vi "Custom Drive.vi"(8 "error in (no error)":errorcluster, 9 "RightSpeed":dbl, 10 "LeftSpeed":dbl, 11 "RobotDriveDevRef":T1={"DevStatus"={"status"=FALSE, "code"=0, "source"=""}, "Motors[]"=[], "Square Inputs"=FALSE, "Max Output"=1.0}) -> (0 "error out":errorcluster, 2 "Motor Values":dbl[](array[numeric]), 3 "RobotDriveDevRef":T1={"DevStatus"={"status"=FALSE, "code"=0, "source"=""}, "Motors[]"=[], "Square Inputs"=FALSE, "Max Output"=1.0})   [LabVIEW 2015]
doc: "Determines the motor configuration and sends the speed values to the appropriate motors.\n\nThis software is licensed. Open the labview\\readme\\WPI Robotics Library Open Source License.txt file for more information."
uses:
  <vilib>/Rock Robotics/WPI/RobotDrive/WPI_RobotDriveDevRef.ctl
  <vilib>/Rock Robotics/WPI/MotorControl/WPI_MotorControlDeviceRef.ctl
  <vilib>/Rock Robotics/WPI/MotorControl/WPI_MotorControlType.ctl
  <vilib>/Rock Robotics/SystemInterfaces/DIO/FPGA_DIOPWMChannel.ctl
  <vilib>/Rock Robotics/WPI/PWM/WPI_PWMDeadband.ctl
  <vilib>/Rock Robotics/WPI/CAN/Jaguar/SubVIs/WPI_CANJaguar_ControlMode.ctl
  <vilib>/Rock Robotics/WPI/CAN/TalonSRX/WPI_CANTalonSRX_APIControlMode.ctl
  <vilib>/Rock Robotics/WPI/RobotDrive/WPI_RobotDriveSafetyCheck.vi
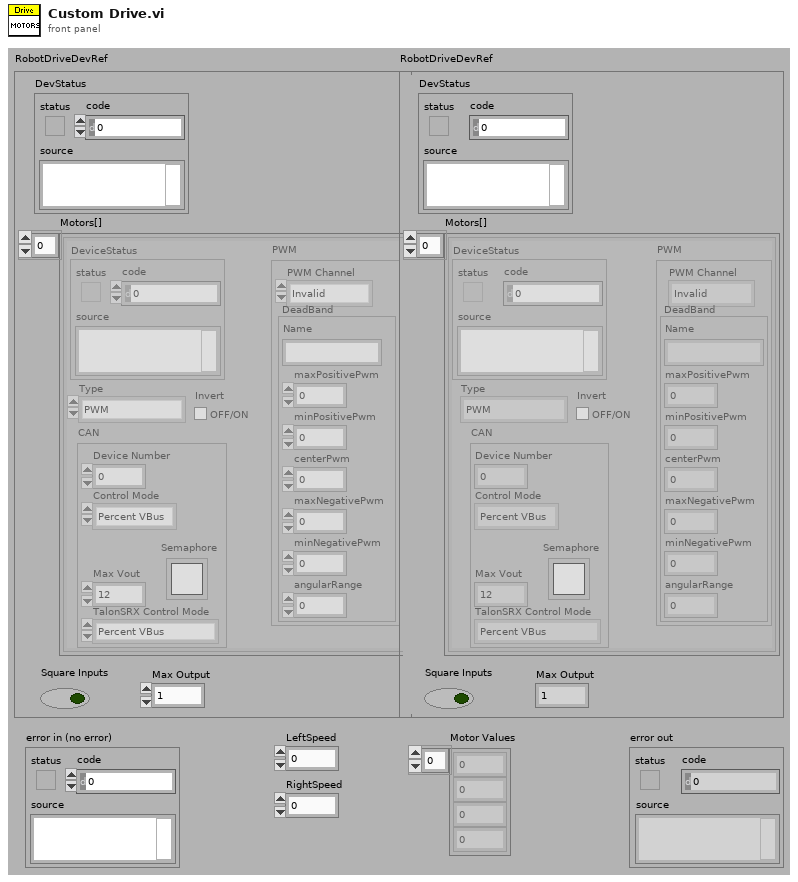
[diagram p1: front panel]
types:
  T1 = typedef "WPI_RobotDriveDevRef.ctl" = cluster{"DevStatus":errorcluster, "Motors[]":T2[], "Square Inputs":bool, "Max Output":dbl}
  T2 = typedef "WPI_MotorControlDeviceRef.ctl" = cluster{"DeviceStatus":errorcluster, "Type":T3, "PWM":cluster{"PWM Channel":T4, "DeadBand":T5}, "CAN":cluster{"Device Number":u8, "Control Mode":T6, "Semaphore":T7, "Max Vout":dbl, "TalonSRX Control Mode":T8}, "Invert":bool}
  T3 = typedef "WPI_MotorControlType.ctl" = enum16{"PWM", "CAN", "CANTalonSRX"}
  T4 = typedef "FPGA_DIOPWMChannel.ctl" = enum8{"PWM 0", "PWM 1", "PWM 2", "PWM 3", "PWM 4", "PWM 5", "PWM 6", "PWM 7", "PWM 8", "PWM 9", "PWM MXP 0", "PWM MXP 1", "PWM MXP 2", "PWM MXP 3", "PWM MXP 4", "PWM MXP 5", "PWM MXP 6", "PWM MXP 7", "PWM MXP 8", "PWM MXP 9", "Invalid"}
  T5 = typedef "WPI_PWMDeadband.ctl" = cluster{"Name":string, "maxPositivePwm":i32, "minPositivePwm":i32, "centerPwm":i32, "maxNegativePwm":i32, "minNegativePwm":i32, "angularRange":u16}
  T6 = typedef "WPI_CANJaguar_ControlMode.ctl" = enum8{"Percent VBus", "Current", "Speed", "Position", "Voltage"}
  T7 = typedef "Semaphore RefNum" = refnum<k1>
  T8 = typedef "WPI_CANTalonSRX_APIControlMode.ctl" = enum8{"Percent VBus", "Speed", "Position", "Slave", "Unchanged / Invalid", "Voltage Compensation", "Current", "Motion Profile"}
  T9 = enum16{"Rear Left Motor", "Rear Right Motor", "Front Left Motor", "Front Right Motor", "Middle Right Motor", "Middle Left Motor"}
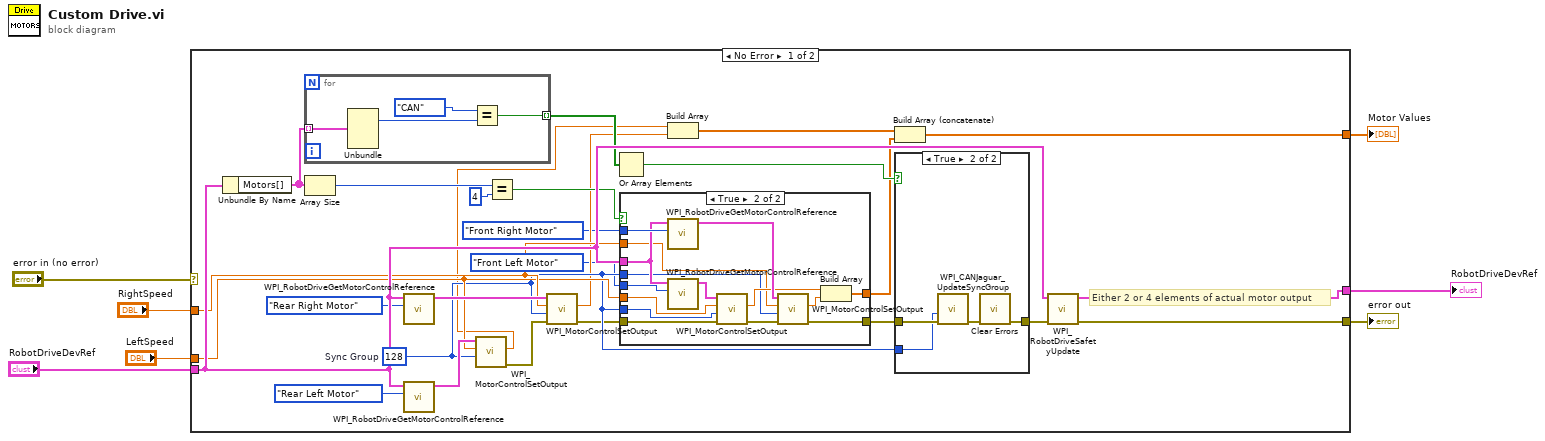
[diagram p0: block diagram]
diagram:
  n1 = case shown="No Error" "error in (no error)" {
    selector: "error in (no error)" -> [_ w61]
    tunnel: "RobotDriveDevRef" -> [w30 w60]
    tunnel: [w12 w60] -> w6
    tunnel: "LeftSpeed" -> [w28 _]
    tunnel: "RightSpeed" -> [w29 _]
    tunnel: [w13 w61] -> w2
    tunnel: [w15 _] -> w1
    frame No Error {
      w26 = u8 128  # Sync Group
      # "Either 2 or 4 elements of actual motor output"
      n2 = Unbundle By Name(w30) -> ("Motors[]"=w25:T2[])
      n3 = for {
        tunnel: w25 -> [w38] mode=indexing
        tunnel: [w35] -> w24 mode=indexing
        n4 = Unbundle(w38) -> ("Type"=w37:T3)  [unwired: 4 out]
        n5 = Equal?(x=enum16{"PWM", "CAN"}."CAN" ("Type"), y=w37) -> (x = y?=w35:bool)
      }
      n6 = Array Size(array=w25) -> (size(s)=w34:i32)
      n7 = call <vilib>:"WPI_RobotDriveGetMotorControlReference.vi"("MotorIndex"=T9."Rear Right Motor", "RobotDriveDevRef"=w30) -> ("MotorControlDeviceRef"=w32:T2)  [unwired: 9 out]
      n8 = call <vilib>:"WPI_RobotDriveGetMotorControlReference.vi"("MotorIndex"=T9."Rear Left Motor", "RobotDriveDevRef"=w30) -> ("MotorControlDeviceRef"=w31:T2)  [unwired: 9 out]
      n9 = call <vilib>:"WPI_MotorControlSetOutput.vi"("Sync Group / Parameter Slot"=w26, "Output"=w28, "MotorControlDevRef"=w31) -> ("error out"=w22:errorcluster, "Motor Output"=w19:dbl)  [unwired: 2 in, 5 out]
      n10 = Equal?(x=w34, y=4) -> (x = y?=w27:bool)
      n11 = call <vilib>:"WPI_MotorControlSetOutput.vi"("error in (no error)"=w22, "Sync Group / Parameter Slot"=w26, "Output"=w29, "MotorControlDevRef"=w32) -> ("error out"=w20:errorcluster, "Motor Output"=w18:dbl)  [unwired: 1 in, 5 out]
      n12 = Or Array Elements(Boolean array=w24) -> (logical OR=w23:bool)
      n13 = case shown="True" w27 {
        tunnel: T9."Front Left Motor" -> [_ w59]
        tunnel: T9."Front Right Motor" -> [_ w58]
        tunnel: w30 -> [_ w49]
        tunnel: w26 -> [_ w48]
        tunnel: w29 -> [_ w47]
        tunnel: w28 -> [_ w46]
        tunnel: [w44 w45] -> w21
        tunnel: w26 -> [_ w55]
        tunnel: w20 -> [w44 w53]
        tunnel: [_ w50] -> w17
        frame False {
        }
        frame True {
          n14 = call <vilib>:"WPI_RobotDriveGetMotorControlReference.vi"("MotorIndex"=w58, "RobotDriveDevRef"=w49) -> ("MotorControlDeviceRef"=w57:T2)  [unwired: 9 out]
          n15 = call <vilib>:"WPI_RobotDriveGetMotorControlReference.vi"("MotorIndex"=w59, "RobotDriveDevRef"=w49) -> ("MotorControlDeviceRef"=w56:T2)  [unwired: 9 out]
          n16 = call <vilib>:"WPI_MotorControlSetOutput.vi"("error in (no error)"=w53, "Sync Group / Parameter Slot"=w55, "Output"=w46, "MotorControlDevRef"=w56) -> ("error out"=w54:errorcluster, "Motor Output"=w51:dbl)  [unwired: 1 in, 5 out]
          n17 = call <vilib>:"WPI_MotorControlSetOutput.vi"("error in (no error)"=w54, "Sync Group / Parameter Slot"=w48, "Output"=w47, "MotorControlDevRef"=w57) -> ("error out"=w45:errorcluster, "Motor Output"=w52:dbl)  [unwired: 1 in, 5 out]
          n18 = Build Array(w51, w52) -> (w50:dbl[])
        }
      }
      n19 = Build Array(w19, w18) -> (w16:dbl[])
      n20 = Build Array (concatenate)(w16, w17) -> (w15:dbl[])
      n21 = case shown="True" w23 {
        tunnel: w21 -> [w39 w42]
        tunnel: w26 -> [_ w41]
        tunnel: [w39 w40] -> w14
        frame False {
        }
        frame True {
          n22 = call <vilib>:"WPI_CANJaguar_UpdateSyncGroup.vi"("error in (no error)"=w42, "Sync Group"=w41) -> ("error out"=w43:errorcluster)  [unwired: 9 out]
          n23 = call <vilib>:"Clear Errors.vi"("error in (no error)"=w43) -> ("error out"=w40:errorcluster)  [unwired: 1 in, 5 out]
        }
      }
      n24 = call <vilib>:"WPI_RobotDriveSafetyUpdate.vi"("error in (no error)"=w14, "RobotDriveDevRef"=w30) -> ("error out"=w13:errorcluster, "RobotDriveDevRef"=w12:T1)  [unwired: 8 out]
    }
    frame Error {
    }
  }
  "RobotDriveDevRef" <- w6
  "error out" <- w2
  "Motor Values" <- w1
